vi "pos_motor2displayunit.vi"(8 "error in (no error)":errorcluster, 10 "pos in motor (pulses)":dbl, 11 "Motor in":refnum<class "Motor.lvclass">) -> (0 "error out":errorcluster, 2 "pos in display unit":dbl, 3 "Motor out":refnum<class "Motor.lvclass">)   [LabVIEW 2016, in "Hardware.lvlib" / "Motor.lvlib" / "Motor.lvclass"]
uses:
  <userlib>/Common Components/Hardware/Motor/Motor/Motor.lvclass
  <userlib>/Common Components/Hardware/Motor/Motor/Motor.lvclass/Motor.ctl
  <userlib>/Common Components/Hardware/Motor/Motor/Accessor/Read unit mode.vi
  <userlib>/Common Components/Hardware/Motor/Motor/Accessor/Read motor pulses per revolution.vi
  <userlib>/Common Components/Hardware/Motor/Motor/Accessor/Read display units per motor rev.vi
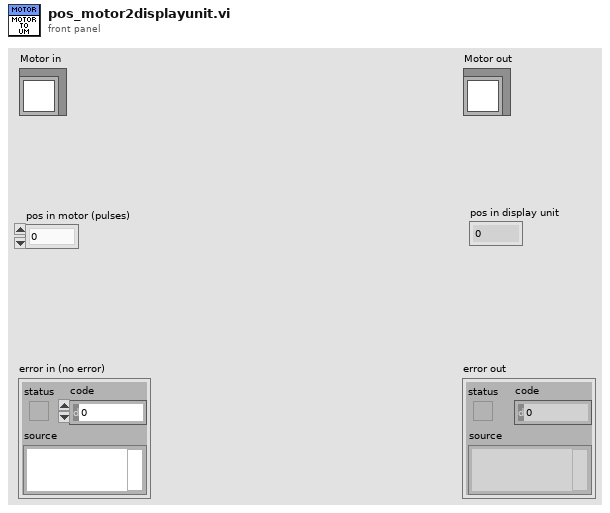
[diagram p1: front panel]
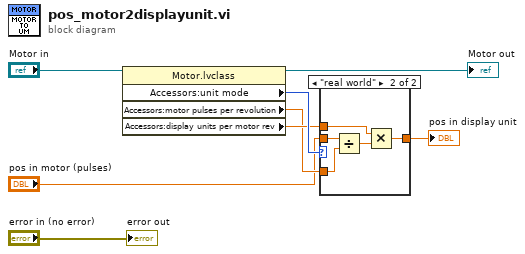
[diagram p0: block diagram]
diagram:
  n1 = property class="Motor.lvclass"(reference="Motor in") -> (reference out=→"Motor out":refnum<class "Motor.lvclass">, "Accessors:unit mode"=w5:enum16{"motor pulses", "real world"}, "Accessors:motor pulses per revolution"=w3:dbl, "Accessors:display units per motor rev"=w4:dbl)  [unwired: 1 in, 1 out]
  n2 = case shown="\"real world\"" w5 {
    tunnel: [w9 w12] -> w1
    tunnel: "pos in motor (pulses)" -> [w9 w14]
    tunnel: w4 -> [_ w10]
    tunnel: w3 -> [_ w11]
    frame "motor pulses", Default {
    }
    frame "real world" {
      n3 = Divide(x=w14, y=w11) -> (x/y=w13:dbl)
      n4 = Multiply(x=w10, y=w13) -> (x*y=w12:dbl)
    }
  }
  "pos in display unit" <- w1
  "error out" <- "error in (no error)"
